vi "Auto Show Hide.vi"(8 "error in (no error)":errorcluster, 11 "Fault Monitor in":refnum<class "Fault Monitor.lvclass">) -> (0 "error out":errorcluster, 3 "Fault Monitor out":refnum<class "Fault Monitor.lvclass">)   [LabVIEW 2023, in "Fault Monitor.lvlib" / "Fault Monitor.lvclass"]
uses:
  Library/Fault Monitor.lvclass
  Library/Fault Monitor.lvclass/Fault Monitor.ctl
  builds/Framework/Engine.lvlibp/Engine/Accessors/Read Self Q.vi
  builds/Framework/Actor Framework.lvlibp/1abvi3w/vi.lib/ActorFramework/Message Enqueuer/Message Enqueuer.lvclass
  builds/Main/Docking.lvlibp/Docking Messages/Adjust Splitter Msg/Adjust Splitter Msg.lvclass
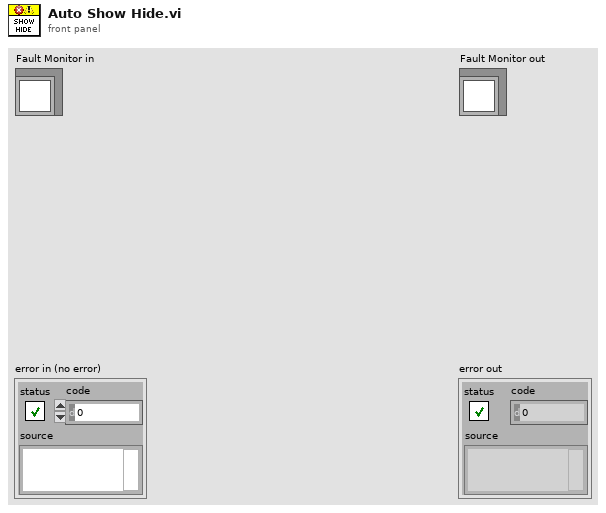
[diagram p1: front panel]
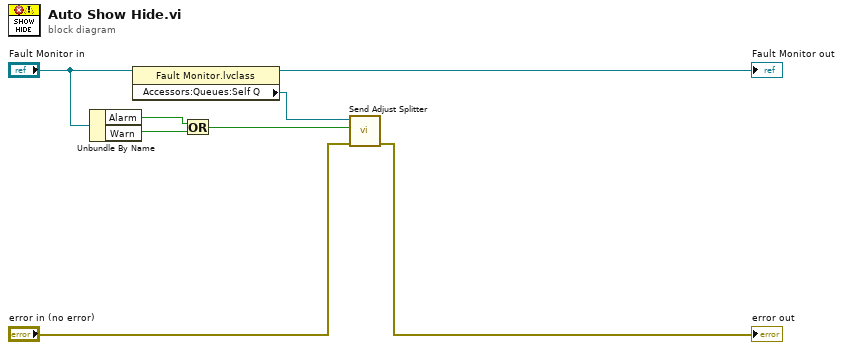
[diagram p0: block diagram]
diagram:
  n1 = Unbundle By Name("Fault Monitor in") -> ("Alarm"=w7:bool, "Warn"=w6:bool)
  n2 = property class="Fault Monitor.lvclass"(reference="Fault Monitor in") -> (reference out=→"Fault Monitor out":refnum<class "Fault Monitor.lvclass">, "Accessors:Queues:Self Q"=w4:refnum<class "Message Enqueuer.lvclass">)  [unwired: 1 in, 1 out]
  n3 = Or(x=w7, y=w6) -> (x .or. y?=w1:bool)
  n4 = call "Send Adjust Splitter.vi"("error in (no error)"="error in (no error)", "Show"=w1, "Message Enqueuer"=w4) -> ("error out"=→"error out":errorcluster)  [unwired: 7 in, 1 out]
